vi "FinsManager_main.vi"(8 "Error In":errorcluster) -> (0 "Error Out":errorcluster)   [LabVIEW 2013]
uses:
  My Computer/Controls/Fin Arrangement.ctl
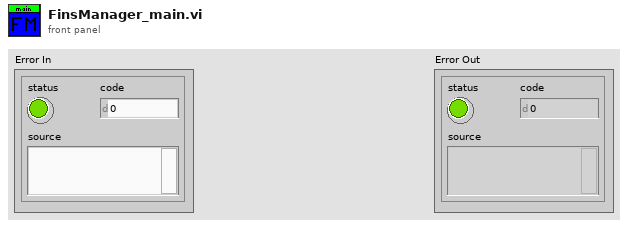
[diagram p1: front panel]
types:
  T1 = typedef "Fin Arrangement.ctl" = cluster{"Fin0":u8, "Fin3":u8, "Fin1":u8, "Fin2":u8}
  T2 = cluster{"Fin0":u8, "Fin1":u8, "Fin2":u8, "Fin3":u8}
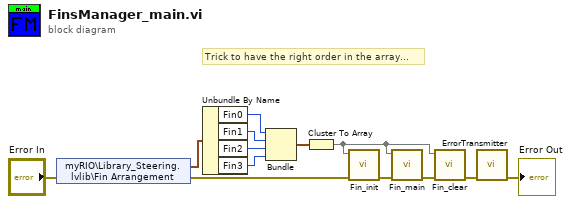
[diagram p0: block diagram]
diagram:
  # "Trick to have the right order in the array..."
  n1 = shared-variable "myRIO\\Library_Steering.lvlib\\Fin Arrangement"(error in="Error In") -> (w13:T1, error out=w5:errorcluster)
  n2 = Unbundle By Name(w13) -> ("Fin0"=w12:u8, "Fin1"=w11:u8, "Fin2"=w10:u8, "Fin3"=w9:u8)
  n3 = Bundle("Fin0"=w12, "Fin1"=w11, "Fin2"=w10, "Fin3"=w9) -> (w8:T2)  [unwired: 1 in]
  n4 = Cluster To Array(cluster=w8) -> (array=w7:u8[])
  n5 = call "Fin_init.vi"("Error In"=w5, "Fin Arrangement (SORTED)"=w7) -> ("Error Out"=w4:errorcluster)  [unwired: 9 in]
  n6 = call "Fin_main.vi"("Error In"=w4, "Fin Arrangement (SORTED)"=w7) -> ("Error Out"=w3:errorcluster)  [unwired: 9 in]
  n7 = call "Fin_clear.vi"("Error In"=w3, "Fin Arrangement (SORTED)"=w7) -> ("Error Out"=w2:errorcluster)  [unwired: 9 in]
  n8 = call "ErrorTransmitter.vi"("Error In"=w2) -> ("Error Out"=→"Error Out":errorcluster)  [unwired: 10 in]
